vi "Lichen Analysis.vi"(0 "Parameters (Rejilla)":T2(array[cluster])=[{"Name"="Rectangle 1", "Type"=enum."Rotated Rectangle", "Coordinates"=[0, 0, 80, 76, 0], "Colors"=[16711680], "Drawing Mode"=0, "Text"="Your Text", "Results"=[], "Font, Size & Style"={"Desired Font (Application)"=enum."System Font", "[User-specified Font]"={"Font Name"="Tahoma", "Size"=13, "Strikeout?"=FALSE, "Italic?"=FALSE, "Underline?"=FALSE, "Outline?"=FALSE, "Shadow?"=FALSE, "Bold?"=FALSE, "Rotation Angle"=0.0}, "Horizontal Alignment"=0, "Vertical Alignment"=0}, "Image File Path"=path "", "Use Keying Color"=FALSE}, {"Name"="Rectangle 2", "Type"=enum."Rotated Rectangle", "Coordinates"=[81, 0, 161, 76, 0], "Colors"=[16717824], "Drawing Mode"=0, "Text"="Your Text", "Results"=[], "Font, Size & Style"={"Desired Font (Application)"=enum."System Font", "[User-specified Font]"={"Font Name"="Tahoma", "Size"=13, "Strikeout?"=FALSE, "Italic?"=FALSE, "Underline?"=FALSE, "Outline?"=FALSE, "Shadow?"=FALSE, "Bold?"=FALSE, "Rotation Angle"=0.0}, "Horizontal Alignment"=0, "Vertical Alignment"=0}, "Image File Path"=path "", "Use Keying Color"=FALSE}, {"Name"="Rectangle 3", "Type"=enum."Rotated Rectangle", "Coordinates"=[0, 77, 80, 152, 0], "Colors"=[16717824], "Drawing Mode"=0, "Text"="Your Text", "Results"=[], "Font, Size & Style"={"Desired Font (Application)"=enum."System Font", "[User-specified Font]"={"Font Name"="Tahoma", "Size"=13, "Strikeout?"=FALSE, "Italic?"=FALSE, "Underline?"=FALSE, "Outline?"=FALSE, "Shadow?"=FALSE, "Bold?"=FALSE, "Rotation Angle"=0.0}, "Horizontal Alignment"=0, "Vertical Alignment"=0}, "Image File Path"=path "", "Use Keying Color"=FALSE}, {"Name"="Rectangle 4", "Type"=enum."Rotated Rectangle", "Coordinates"=[81, 77, 161, 152, 0], "Colors"=[16717824], "Drawing Mode"=0, "Text"="Your Text", "Results"=[], "Font, Size & Style"={"Desired Font (Application)"=enum."System Font", "[User-specified Font]"={"Font Name"="Tahoma", "Size"=13, "Strikeout?"=FALSE, "Italic?"=FALSE, "Underline?"=FALSE, "Outline?"=FALSE, "Shadow?"=FALSE, "Bold?"=FALSE, "Rotation Angle"=0.0}, "Horizontal Alignment"=0, "Vertical Alignment"=0}, "Image File Path"=path "", "Use Keying Color"=FALSE}, {"Name"="Rectangle 5", "Type"=enum."Rotated Rectangle", "Coordinates"=[0, 153, 80, 228, 0], "Colors"=[16717824], "Drawing Mode"=0, "Text"="Your Text", "Results"=[], "Font, Size & Style"={"Desired Font (Application)"=enum."System Font", "[User-specified Font]"={"Font Name"="Tahoma", "Size"=13, "Strikeout?"=FALSE, "Italic?"=FALSE, "Underline?"=FALSE, "Outline?"=FALSE, "Shadow?"=FALSE, "Bold?"=FALSE, "Rotation Angle"=0.0}, "Horizontal Alignment"=0, "Vertical Alignment"=0}, "Image File Path"=path "", "Use Keying Color"=FALSE}, {"Name"="Rectangle 6", "Type"=enum."Rotated Rectangle", "Coordinates"=[81, 153, 161, 228, 0], "Colors"=[16717824], "Drawing Mode"=0, "Text"="Your Text", "Results"=[], "Font, Size & Style"={"Desired Font (Application)"=enum."System Font", "[User-specified Font]"={"Font Name"="Tahoma", "Size"=13, "Strikeout?"=FALSE, "Italic?"=FALSE, "Underline?"=FALSE, "Outline?"=FALSE, "Shadow?"=FALSE, "Bold?"=FALSE, "Rotation Angle"=0.0}, "Horizontal Alignment"=0, "Vertical Alignment"=0}, "Image File Path"=path "", "Use Keying Color"=FALSE}, {"Name"="Text 1", "Type"=enum."Text", "Coordinates"=[3, 73], "Colors"=[2817810, 16777216], "Drawing Mode"=0, "Text"="Cell 1", "Results"=[], "Font, Size & Style"={"Desired Font (Application)"=enum."System Font", "[User-specified Font]"={"Font Name"="Tahoma", "Size"=13, "Strikeout?"=FALSE, "Italic?"=FALSE, "Underline?"=FALSE, "Outline?"=FALSE, "Shadow?"=FALSE, "Bold?"=FALSE, "Rotation Angle"=0.0}, "Horizontal Alignment"=0, "Vertical Alignment"=0}, "Image File Path"=path "", "Use Keying Color"=FALSE}, {"Name"="Text 2", "Type"=enum."Text", "Coordinates"=[83, 73], "Colors"=[2817810, 16777216], "Drawing Mode"=0, "Text"="Cell 2", "Results"=[], "Font, Size & Style"={"Desired Font (Application)"=enum."System Font", "[User-specified Font]"={"Font Name"="Tahoma", "Size"=13, "Strikeout?"=FALSE, "Italic?"=FALSE, "Underline?"=FALSE, "Outline?"=FALSE, "Shadow?"=FALSE, "Bold?"=FALSE, "Rotation Angle"=0.0}, "Horizontal Alignment"=0, "Vertical Alignment"=0}, "Image File Path"=path "", "Use Keying Color"=FALSE}, {"Name"="Text 3", "Type"=enum."Text", "Coordinates"=[3, 149], "Colors"=[2817810, 16777216], "Drawing Mode"=0, "Text"="Cell 3", "Results"=[], "Font, Size & Style"={"Desired Font (Application)"=enum."System Font", "[User-specified Font]"={"Font Name"="Tahoma", "Size"=13, "Strikeout?"=FALSE, "Italic?"=FALSE, "Underline?"=FALSE, "Outline?"=FALSE, "Shadow?"=FALSE, "Bold?"=FALSE, "Rotation Angle"=0.0}, "Horizontal Alignment"=0, "Vertical Alignment"=0}, "Image File Path"=path "", "Use Keying Color"=FALSE}, {"Name"="Text 4", "Type"=enum."Text", "Coordinates"=[83, 149], "Colors"=[2817810, 16777216], "Drawing Mode"=0, "Text"="Cell 4", "Results"=[], "Font, Size & Style"={"Desired Font (Application)"=enum."System Font", "[User-specified Font]"={"Font Name"="Tahoma", "Size"=13, "Strikeout?"=FALSE, "Italic?"=FALSE, "Underline?"=FALSE, "Outline?"=FALSE, "Shadow?"=FALSE, "Bold?"=FALSE, "Rotation Angle"=0.0}, "Horizontal Alignment"=0, "Vertical Alignment"=0}, "Image File Path"=path "", "Use Keying Color"=FALSE}, {"Name"="Text 5", "Type"=enum."Text", "Coordinates"=[3, 225], "Colors"=[2817810, 16777216], "Drawing Mode"=0, "Text"="Cell 5", "Results"=[], "Font, Size & Style"={"Desired Font (Application)"=enum."System Font", "[User-specified Font]"={"Font Name"="Tahoma", "Size"=13, "Strikeout?"=FALSE, "Italic?"=FALSE, "Underline?"=FALSE, "Outline?"=FALSE, "Shadow?"=FALSE, "Bold?"=FALSE, "Rotation Angle"=0.0}, "Horizontal Alignment"=0, "Vertical Alignment"=0}, "Image File Path"=path "", "Use Keying Color"=FALSE}, {"Name"="Text 6", "Type"=enum."Text", "Coordinates"=[83, 225], "Colors"=[65407, 16777216], "Drawing Mode"=0, "Text"="Cell 6", "Results"=[], "Font, Size & Style"={"Desired Font (Application)"=enum."System Font", "[User-specified Font]"={"Font Name"="Tahoma", "Size"=13, "Strikeout?"=FALSE, "Italic?"=FALSE, "Underline?"=FALSE, "Outline?"=FALSE, "Shadow?"=FALSE, "Bold?"=FALSE, "Rotation Angle"=0.0}, "Horizontal Alignment"=0, "Vertical Alignment"=0}, "Image File Path"=path "", "Use Keying Color"=FALSE}] {"Drawing Mode" items=["Frame", "Fill", "Highlight"]; "Results"."String Format" items=["Decimal", "Hexadecimal", "Octal", "Fractional", "Exponential", "Engineering"]; "Font, Size & Style"."Horizontal Alignment" items=["Left", "Center", "Right"]; "Font, Size & Style"."Vertical Alignment" items=["Bottom", "Top", "Baseline"]}, 1 "ROI Descriptor (Lichen 1 Cell 1)":T1={"Global Rectangle"=[1, 0, 80, 76], "Contours"=[{"ID"=enum."External", "Type"=12, "Coordinates"=[1, 0, 80, 76, 0]}]} {"Contours"."Type" items=["No Selection", "Point", "Line", "Rectangle", "Oval", "Polygon", "Freehand Region", "Annulus", "Unused2", "Unused3", "Broken Line", "Freehand Line", "Rotated Rectangle"]}, 2 "ROI Descriptor (Lichen 1 Cell 2)":T1={"Global Rectangle"=[81, 0, 161, 76], "Contours"=[{"ID"=enum."External", "Type"=12, "Coordinates"=[81, 0, 161, 76, 0]}]} {"Contours"."Type" items=["No Selection", "Point", "Line", "Rectangle", "Oval", "Polygon", "Freehand Region", "Annulus", "Unused2", "Unused3", "Broken Line", "Freehand Line", "Rotated Rectangle"]}, 3 "ROI Descriptor (Lichen 1 Cell 3)":T1={"Global Rectangle"=[0, 77, 80, 152], "Contours"=[{"ID"=enum."External", "Type"=12, "Coordinates"=[0, 77, 80, 152, 0]}]} {"Contours"."Type" items=["No Selection", "Point", "Line", "Rectangle", "Oval", "Polygon", "Freehand Region", "Annulus", "Unused2", "Unused3", "Broken Line", "Freehand Line", "Rotated Rectangle"]}, 4 "ROI Descriptor (Lichen 1 Cell 4)":T1={"Global Rectangle"=[81, 77, 161, 152], "Contours"=[{"ID"=enum."External", "Type"=12, "Coordinates"=[81, 77, 161, 152, 0]}]} {"Contours"."Type" items=["No Selection", "Point", "Line", "Rectangle", "Oval", "Polygon", "Freehand Region", "Annulus", "Unused2", "Unused3", "Broken Line", "Freehand Line", "Rotated Rectangle"]}, 5 "ROI Descriptor (Lichen 1 Cell 5)":T1={"Global Rectangle"=[0, 153, 80, 228], "Contours"=[{"ID"=enum."External", "Type"=12, "Coordinates"=[0, 153, 80, 228, 0]}]} {"Contours"."Type" items=["No Selection", "Point", "Line", "Rectangle", "Oval", "Polygon", "Freehand Region", "Annulus", "Unused2", "Unused3", "Broken Line", "Freehand Line", "Rotated Rectangle"]}, 6 "ROI Descriptor (Lichen 1 Cell 6)":T1={"Global Rectangle"=[81, 153, 161, 228], "Contours"=[{"ID"=enum."External", "Type"=12, "Coordinates"=[81, 153, 161, 228, 0]}]} {"Contours"."Type" items=["No Selection", "Point", "Line", "Rectangle", "Oval", "Polygon", "Freehand Region", "Annulus", "Unused2", "Unused3", "Broken Line", "Freehand Line", "Rotated Rectangle"]}, 7 "error in":errorcluster, 8 "ROI Descriptor (Lichen 2 Cell1)":T1={"Global Rectangle"=[0, 0, 80, 76], "Contours"=[{"ID"=enum."External", "Type"=12, "Coordinates"=[0, 0, 80, 76, 0]}]} {"Contours"."Type" items=["No Selection", "Point", "Line", "Rectangle", "Oval", "Polygon", "Freehand Region", "Annulus", "Unused2", "Unused3", "Broken Line", "Freehand Line", "Rotated Rectangle"]}, 9 "ROI Descriptor (Lichen 2 Cell 2)":T1={"Global Rectangle"=[81, 0, 161, 76], "Contours"=[{"ID"=enum."External", "Type"=12, "Coordinates"=[81, 0, 161, 76, 0]}]} {"Contours"."Type" items=["No Selection", "Point", "Line", "Rectangle", "Oval", "Polygon", "Freehand Region", "Annulus", "Unused2", "Unused3", "Broken Line", "Freehand Line", "Rotated Rectangle"]}, 10 "ROI Descriptor (Lichen 2 Cell 3)":T1={"Global Rectangle"=[0, 77, 80, 152], "Contours"=[{"ID"=enum."External", "Type"=12, "Coordinates"=[0, 77, 80, 152, 0]}]} {"Contours"."Type" items=["No Selection", "Point", "Line", "Rectangle", "Oval", "Polygon", "Freehand Region", "Annulus", "Unused2", "Unused3", "Broken Line", "Freehand Line", "Rotated Rectangle"]}, 11 "ROI Descriptor (Lichen 2 Cell 4)":T1={"Global Rectangle"=[81, 77, 161, 152], "Contours"=[{"ID"=enum."External", "Type"=12, "Coordinates"=[81, 77, 161, 152, 0]}]} {"Contours"."Type" items=["No Selection", "Point", "Line", "Rectangle", "Oval", "Polygon", "Freehand Region", "Annulus", "Unused2", "Unused3", "Broken Line", "Freehand Line", "Rotated Rectangle"]}, 12 "ROI Descriptor (Lichen 2 Cell 5)":T1={"Global Rectangle"=[0, 153, 80, 228], "Contours"=[{"ID"=enum."External", "Type"=12, "Coordinates"=[0, 153, 80, 228, 0]}]} {"Contours"."Type" items=["No Selection", "Point", "Line", "Rectangle", "Oval", "Polygon", "Freehand Region", "Annulus", "Unused2", "Unused3", "Broken Line", "Freehand Line", "Rotated Rectangle"]}, 13 "ROI Descriptor (Lichen 2 Cell 6)":T1={"Global Rectangle"=[81, 153, 161, 228], "Contours"=[{"ID"=enum."External", "Type"=12, "Coordinates"=[81, 153, 161, 228, 0]}]} {"Contours"."Type" items=["No Selection", "Point", "Line", "Rectangle", "Oval", "Polygon", "Freehand Region", "Annulus", "Unused2", "Unused3", "Broken Line", "Freehand Line", "Rotated Rectangle"]}) -> (14 "Histogram (Histogram 2)":u32[][](array[numeric]), 15 "Number of Matches (Lichen 2 Cell 6)":i32, 16 "Number of Matches (Lichen 2 Cell 5)":i32, 17 "Number of Matches (Lichen 2 Cell 4)":i32, 18 "Number of Matches (Lichen 2 Cell 3)":i32, 19 "Number of Matches (Lichen 2 Cell 2)":i32, 20 "Number of Matches (Lichen 1 Cell 1)":i32, 21 "Number of Matches (Lichen 1 Cell 2)":i32, 22 "Number of Matches (Lichen 1 Cell 3)":i32, 23 "Number of Matches (Lichen 1 Cell 4)":i32, 24 "Number of Matches (Lichen 1 Cell 5)":i32, 25 "Number of Matches (Lichen 1 Cell 6)":i32, 26 "Number of Matches (Lichen 2 Cell1)":i32, 27 "error out":errorcluster)   [LabVIEW 2018]
uses:
  <vilib>/vision/NI_Vision_Development_Module.lvlib
panel:
  out "Image Out":T3(plugin-control)
  out "Histogram Graph 2":u32[][](graph)
  out "Histogram Graph":u32[][](graph)
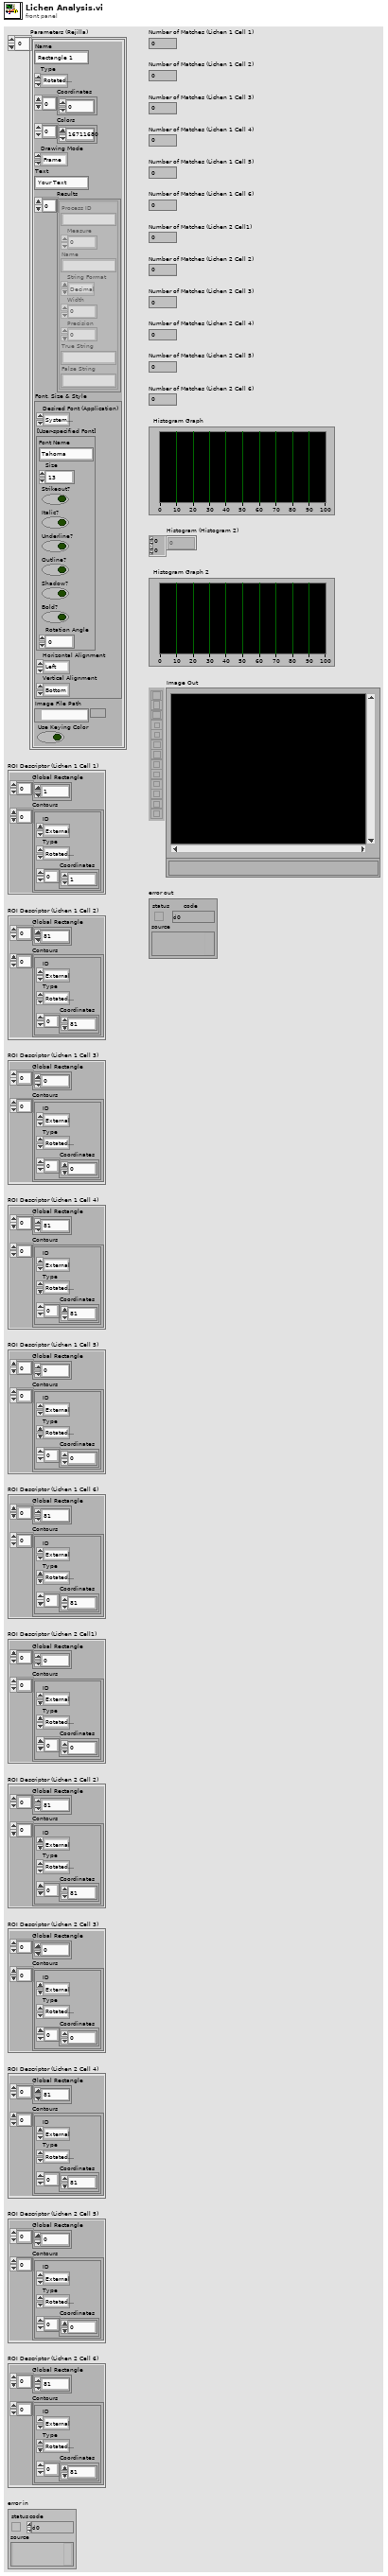
[diagram p1: front panel]
types:
  T1 = cluster{"Global Rectangle":i32[], "Contours":cluster{"ID":enum32{"External", "Internal"}, "Type":u32, "Coordinates":i32[]}[]}
  T2 = cluster{"Name":string, "Type":enum16{"Line", "Broken Line", "Free Hand Line", "Rotated Rectangle", "Oval", "Polygon", "Free Hand", "Bitmap", "Text"}, "Coordinates":i32[], "Colors":u32[], "Drawing Mode":u32, "Text":string, "Results":cluster{"Process ID":string, "Measure":u16, "Name":string, "String Format":u16, "Width":i16, "Precision":i16, "True String":string, "False String":string}[], "Font, Size & Style":cluster{"Desired Font (Application)":enum16{"User-specified Font", "Application Font", "System Font", "Dialog Font"}, "[User-specified Font]":cluster{"Font Name":string, "Size":i16, "Strikeout?":bool, "Italic?":bool, "Underline?":bool, "Outline?":bool, "Shadow?":bool, "Bold?":bool, "Rotation Angle":dbl}, "Horizontal Alignment":i16, "Vertical Alignment":i16}, "Image File Path":path, "Use Keying Color":bool}[]
  T3 = typedef "IMAQ Image.ctl" = refnum<image>
  T4 = typedef "Image Type" = u32
  T5 = cluster{"Position":cluster{"x":sgl, "y":sgl}, "Angle":sgl, "Scale":sgl, "Score":sgl, "Bounding Box":cluster{"x":sgl, "y":sgl}[]}[]
diagram:
  w1 = u32 1 items=["Grayscale", "Binary", "Gradient", "Rainbow", "Temperature", "User Defined", "Binary 16 Bit", "Gradient 16 Bit", "Rainbow 16 Bit", "Temperature 16 Bit", "User Defined 16 Bit"] ("Palette Type")
  w10 = u16 0 items=["RGB", "HSL", "HSV", "HSI"] ("Color Mode")
  w8 = T1 {"Global Rectangle"=[-10, 0, 161, 234], "Contours"=[{"ID"=enum."External", "Type"=3, "Coordinates"=[-10, 0, 161, 234]}]}  # ROI Descriptor
  w18 = u16 1 items=["RGB", "HSL", "HSV", "HSI"] ("Color Mode")
  w27 = 10  # Bit Depth
  w28 = FALSE  # Set Bit Depth
  w37 = u16 0 items=["RGB", "HSL", "HSV", "HSI"] ("Color Mode")
  w35 = T1 {"Global Rectangle"=[0, 0, 161, 228], "Contours"=[{"ID"=enum."External", "Type"=3, "Coordinates"=[0, 0, 161, 228]}]}  # ROI Descriptor
  w54 = u16 0 items=["RGB", "HSL", "HSV", "HSI"] ("Color Mode")
  w63 = "Lichen 2 Cell 6" ("Step Name")
  w68 = T4 4 items=["Grayscale (U8)", "Grayscale (I16)", "Grayscale (SGL)", "Complex (CSG)", "RGB (U32)", "HSL (U32)", "RGB (U64)"] ("Image Type")
  w70 = u32 1 items=["Conservative", "Balance", "Aggressive", "Very Aggressive"] ("Search Strategy")
  w71 = u32 0 items=["Low Sensitivity", "Medium Sensitivity", "High Sensitivity"] ("Color Sensitivity")
  w72 = u32 1 items=["Color and Shape", "Color", "Shape"] ("Match Feature Mode")
  w83 = "Lichen 2 Cell 5" ("Step Name")
  w88 = T4 4 items=["Grayscale (U8)", "Grayscale (I16)", "Grayscale (SGL)", "Complex (CSG)", "RGB (U32)", "HSL (U32)", "RGB (U64)"] ("Image Type")
  w90 = u32 1 items=["Conservative", "Balance", "Aggressive", "Very Aggressive"] ("Search Strategy")
  w91 = u32 0 items=["Low Sensitivity", "Medium Sensitivity", "High Sensitivity"] ("Color Sensitivity")
  w92 = u32 1 items=["Color and Shape", "Color", "Shape"] ("Match Feature Mode")
  w103 = "Lichen 2 Cell 4" ("Step Name")
  w108 = T4 4 items=["Grayscale (U8)", "Grayscale (I16)", "Grayscale (SGL)", "Complex (CSG)", "RGB (U32)", "HSL (U32)", "RGB (U64)"] ("Image Type")
  w110 = u32 0 items=["Conservative", "Balance", "Aggressive", "Very Aggressive"] ("Search Strategy")
  w111 = u32 0 items=["Low Sensitivity", "Medium Sensitivity", "High Sensitivity"] ("Color Sensitivity")
  w112 = u32 1 items=["Color and Shape", "Color", "Shape"] ("Match Feature Mode")
  w123 = "Lichen 2 Cell 3" ("Step Name")
  w128 = T4 4 items=["Grayscale (U8)", "Grayscale (I16)", "Grayscale (SGL)", "Complex (CSG)", "RGB (U32)", "HSL (U32)", "RGB (U64)"] ("Image Type")
  w130 = u32 0 items=["Conservative", "Balance", "Aggressive", "Very Aggressive"] ("Search Strategy")
  w131 = u32 0 items=["Low Sensitivity", "Medium Sensitivity", "High Sensitivity"] ("Color Sensitivity")
  w132 = u32 1 items=["Color and Shape", "Color", "Shape"] ("Match Feature Mode")
  w143 = "Lichen 2 Cell 2" ("Step Name")
  w148 = T4 4 items=["Grayscale (U8)", "Grayscale (I16)", "Grayscale (SGL)", "Complex (CSG)", "RGB (U32)", "HSL (U32)", "RGB (U64)"] ("Image Type")
  w150 = u32 2 items=["Conservative", "Balance", "Aggressive", "Very Aggressive"] ("Search Strategy")
  w151 = u32 0 items=["Low Sensitivity", "Medium Sensitivity", "High Sensitivity"] ("Color Sensitivity")
  w152 = u32 1 items=["Color and Shape", "Color", "Shape"] ("Match Feature Mode")
  w163 = "Lichen 2 Cell1" ("Step Name")
  w168 = T4 4 items=["Grayscale (U8)", "Grayscale (I16)", "Grayscale (SGL)", "Complex (CSG)", "RGB (U32)", "HSL (U32)", "RGB (U64)"] ("Image Type")
  w170 = u32 2 items=["Conservative", "Balance", "Aggressive", "Very Aggressive"] ("Search Strategy")
  w171 = u32 0 items=["Low Sensitivity", "Medium Sensitivity", "High Sensitivity"] ("Color Sensitivity")
  w172 = u32 1 items=["Color and Shape", "Color", "Shape"] ("Match Feature Mode")
  w183 = "Lichen 1 Cell 6" ("Step Name")
  w188 = T4 4 items=["Grayscale (U8)", "Grayscale (I16)", "Grayscale (SGL)", "Complex (CSG)", "RGB (U32)", "HSL (U32)", "RGB (U64)"] ("Image Type")
  w190 = u32 0 items=["Conservative", "Balance", "Aggressive", "Very Aggressive"] ("Search Strategy")
  w191 = u32 0 items=["Low Sensitivity", "Medium Sensitivity", "High Sensitivity"] ("Color Sensitivity")
  w192 = u32 1 items=["Color and Shape", "Color", "Shape"] ("Match Feature Mode")
  w203 = "Lichen 1 Cell 5" ("Step Name")
  w208 = T4 4 items=["Grayscale (U8)", "Grayscale (I16)", "Grayscale (SGL)", "Complex (CSG)", "RGB (U32)", "HSL (U32)", "RGB (U64)"] ("Image Type")
  w210 = u32 0 items=["Conservative", "Balance", "Aggressive", "Very Aggressive"] ("Search Strategy")
  w211 = u32 0 items=["Low Sensitivity", "Medium Sensitivity", "High Sensitivity"] ("Color Sensitivity")
  w212 = u32 1 items=["Color and Shape", "Color", "Shape"] ("Match Feature Mode")
  w223 = "Lichen 1 Cell 4" ("Step Name")
  w228 = T4 4 items=["Grayscale (U8)", "Grayscale (I16)", "Grayscale (SGL)", "Complex (CSG)", "RGB (U32)", "HSL (U32)", "RGB (U64)"] ("Image Type")
  w230 = u32 0 items=["Conservative", "Balance", "Aggressive", "Very Aggressive"] ("Search Strategy")
  w231 = u32 0 items=["Low Sensitivity", "Medium Sensitivity", "High Sensitivity"] ("Color Sensitivity")
  w232 = u32 1 items=["Color and Shape", "Color", "Shape"] ("Match Feature Mode")
  w243 = "Lichen 1 Cell 3" ("Step Name")
  w248 = T4 4 items=["Grayscale (U8)", "Grayscale (I16)", "Grayscale (SGL)", "Complex (CSG)", "RGB (U32)", "HSL (U32)", "RGB (U64)"] ("Image Type")
  w250 = u32 0 items=["Conservative", "Balance", "Aggressive", "Very Aggressive"] ("Search Strategy")
  w251 = u32 0 items=["Low Sensitivity", "Medium Sensitivity", "High Sensitivity"] ("Color Sensitivity")
  w252 = u32 1 items=["Color and Shape", "Color", "Shape"] ("Match Feature Mode")
  w263 = "Lichen 1 Cell 2" ("Step Name")
  w268 = T4 4 items=["Grayscale (U8)", "Grayscale (I16)", "Grayscale (SGL)", "Complex (CSG)", "RGB (U32)", "HSL (U32)", "RGB (U64)"] ("Image Type")
  w270 = u32 0 items=["Conservative", "Balance", "Aggressive", "Very Aggressive"] ("Search Strategy")
  w271 = u32 0 items=["Low Sensitivity", "Medium Sensitivity", "High Sensitivity"] ("Color Sensitivity")
  w272 = u32 1 items=["Color and Shape", "Color", "Shape"] ("Match Feature Mode")
  w283 = "Lichen 1 Cell 1" ("Step Name")
  w288 = T4 4 items=["Grayscale (U8)", "Grayscale (I16)", "Grayscale (SGL)", "Complex (CSG)", "RGB (U32)", "HSL (U32)", "RGB (U64)"] ("Image Type")
  w290 = u32 0 items=["Conservative", "Balance", "Aggressive", "Very Aggressive"] ("Search Strategy")
  w291 = u32 0 items=["Low Sensitivity", "Medium Sensitivity", "High Sensitivity"] ("Color Sensitivity")
  w292 = u32 1 items=["Color and Shape", "Color", "Shape"] ("Match Feature Mode")
  w299 = T4 4 items=["Grayscale (U8)", "Grayscale (I16)", "Grayscale (SGL)", "Complex (CSG)", "RGB (U32)", "HSL (U32)", "RGB (U64)", "Grayscale (U16)"] ("Image Type")
  n1 = Call Chain() -> (call chain=w303:string[])
  n2 = Index Array(array=w303) -> (element=w302:string)  [unwired: 1 in]
  n3 = call "File Dialog"("prompt"="Select an image file...") -> ("selected path"=w300:path)  [unwired: 6 in, 8 out]
  n4 = call "IMAQ Create"("Image Name"=w302, "Image Type"=w299, "error in (no error)"="error in") -> ("New Image"=w306:T3, "error out"=w305:errorcluster)  [unwired: 1 in, 1 out]
  n5 = call "IMAQ ReadFile"("File Path"=w300, "error in (no error)"=w305, "Image"=w306) -> ("error out"=w307:errorcluster, "Image Out"=w298:T3)  [unwired: 2 in, 5 out]
  n6 = call <vilib>:"IVA Overlay - Overlay.vi"("error in (no error)"=w307, "Parameters"="Parameters (Rejilla)", "Image In"=w298) -> ("error out"=w297:errorcluster, "Image Out"=w285:T3)  [unwired: 7 out]
  n7 = while {
    shift-right: [w319] -> w279
    shift-left: _ -> [w318]
    tunnel: [w316] -> w278
    tunnel: w297 -> [w315]
    tunnel: path "C:/Users/anton/Desktop/liquenes/lichen1.png" ("File Path") -> [w311]
    tunnel: w288 -> [w314]
    tunnel: w283 -> [w313]
    shift-right: [w311] -> _
    shift-left: _ -> [w312]
    stop <- FALSE continue-if-true
    n8 = First Call?() -> (First Call?: T/F=w310:bool)
    n9 = Not Equal?(x=w312, y=w311) -> (x != y?=w309:bool)
    n10 = Or(x=w309, y=w310) -> (x .or. y?=w308:bool)
    n11 = case shown="True" w308 {
      tunnel: [w321 w334] -> w319
      tunnel: w318 -> [w321 w326]
      tunnel: [w320 w331] -> w316
      tunnel: w315 -> [w320 w325]
      tunnel: w314 -> [_ w330]
      tunnel: w313 -> [_ w327]
      tunnel: w311 -> [_ w323]
      frame False {
      }
      frame True {
        n12 = Call Chain() -> (call chain=w329:string[])
        n13 = stacked-sequence {
          tunnel: w326 -> [w339]
          tunnel: w325 -> [w338]
          tunnel: [w338] -> w324
          tunnel: [w337] -> _
          frame #0 {
            n14 = call "IMAQ Dispose"("Image"=w339) -> ("error out"=w337:errorcluster)  [unwired: 2 in, 3 out]
          }
        }
        n15 = Index Array(array=w329) -> (element=w328:string)  [unwired: 1 in]
        n16 = Format Into String(format string="CL Template %s %s" ("Image Name"), w328, w327) -> (resulting string=w336:string)  [unwired: 2 in, 1 out]
        n17 = call "IMAQ Create"("Image Name"=w336, "Image Type"=w330, "error in (no error)"=w324) -> ("New Image"=w333:T3, "error out"=w332:errorcluster)  [unwired: 1 in, 1 out]
        n18 = call <vilib>:"IVA Get Alternate Path.vi"("Path In"=w323) -> ("Path Out"=w322:path)  [unwired: 10 out]
        n19 = call "IMAQ Read Image And Vision Info"("File Path"=w322, "error in (no error)"=w332, "Image"=w333) -> ("error out"=w331:errorcluster, "Image Out"=w334:T3)  [unwired: 1 in, 6 out]
      }
    }
  }
  n20 = call <vilib>:"IVA Get Alternate Path.vi"("Path In"=path "C:/Users/anton/Desktop/liquenes/test1.jpg" ("File Path")) -> ("Path Out"=w23:path)  [unwired: 10 out]
  n21 = Unbundle By Name("ROI Descriptor (Lichen 1 Cell 1)") -> ("Global Rectangle"=w280:i32[])
  n22 = call "IMAQ Setup Match Color Pattern"("Match Feature Mode"=w292, "error in (no error)"=w278, "Color Sensitivity"=w291, "Search Strategy"=w290) -> ("Match Color Pattern Setup Data"=w282:string, "error out"=w281:errorcluster)  [unwired: 5 in, 5 out]
  n23 = call "IMAQ Match Color Pattern"("Minimum Match Score"=sgl 700.0, "Number of Matches Requested"=1, "Optional Rectangle"=w280, "error in (no error)"=w281, "Match Color Pattern Setup Data"=w282, "Template Image"=w279, "Image"=w285) -> ("error out"=w286:errorcluster, "Number of Matches"=→"Number of Matches (Lichen 1 Cell 1)":i32, "Matches"=w284:T5)  [unwired: 2 out]
  n24 = call <vilib>:"IVA Store Color Location Results.vi"("error in (no error)"=w286, "Matches"=w284, "Step Name"=w283, "Image in"=w285) -> ("error out"=w277:errorcluster, "Image dup"=w265:T3)  [unwired: 6 out]
  n25 = call <vilib>:"IVA Clear Coordsys Errors.vi"("error in (no error)"=w277) -> ("error out"=w276:errorcluster)  [unwired: 10 in]
  n26 = while {
    shift-right: [w351] -> w259
    shift-left: _ -> [w350]
    tunnel: [w348] -> w258
    tunnel: w276 -> [w347]
    tunnel: path "C:/Users/anton/Desktop/liquenes/lichen1.png" ("File Path") -> [w343]
    tunnel: w268 -> [w346]
    tunnel: w263 -> [w345]
    shift-right: [w343] -> _
    shift-left: _ -> [w344]
    stop <- FALSE continue-if-true
    n27 = First Call?() -> (First Call?: T/F=w342:bool)
    n28 = Not Equal?(x=w344, y=w343) -> (x != y?=w341:bool)
    n29 = Or(x=w341, y=w342) -> (x .or. y?=w340:bool)
    n30 = case shown="True" w340 {
      tunnel: [w353 w366] -> w351
      tunnel: w350 -> [w353 w358]
      tunnel: [w352 w363] -> w348
      tunnel: w347 -> [w352 w357]
      tunnel: w346 -> [_ w362]
      tunnel: w345 -> [_ w359]
      tunnel: w343 -> [_ w355]
      frame False {
      }
      frame True {
        n31 = Call Chain() -> (call chain=w361:string[])
        n32 = stacked-sequence {
          tunnel: w358 -> [w371]
          tunnel: w357 -> [w370]
          tunnel: [w370] -> w356
          tunnel: [w369] -> _
          frame #0 {
            n33 = call "IMAQ Dispose"("Image"=w371) -> ("error out"=w369:errorcluster)  [unwired: 2 in, 3 out]
          }
        }
        n34 = Index Array(array=w361) -> (element=w360:string)  [unwired: 1 in]
        n35 = Format Into String(format string="CL Template %s %s" ("Image Name"), w360, w359) -> (resulting string=w368:string)  [unwired: 2 in, 1 out]
        n36 = call "IMAQ Create"("Image Name"=w368, "Image Type"=w362, "error in (no error)"=w356) -> ("New Image"=w365:T3, "error out"=w364:errorcluster)  [unwired: 1 in, 1 out]
        n37 = call <vilib>:"IVA Get Alternate Path.vi"("Path In"=w355) -> ("Path Out"=w354:path)  [unwired: 10 out]
        n38 = call "IMAQ Read Image And Vision Info"("File Path"=w354, "error in (no error)"=w364, "Image"=w365) -> ("error out"=w363:errorcluster, "Image Out"=w366:T3)  [unwired: 1 in, 6 out]
      }
    }
  }
  n39 = Unbundle By Name("ROI Descriptor (Lichen 1 Cell 2)") -> ("Global Rectangle"=w260:i32[])
  n40 = call "IMAQ Setup Match Color Pattern"("Match Feature Mode"=w272, "error in (no error)"=w258, "Color Sensitivity"=w271, "Search Strategy"=w270) -> ("Match Color Pattern Setup Data"=w262:string, "error out"=w261:errorcluster)  [unwired: 5 in, 5 out]
  n41 = call "IMAQ Match Color Pattern"("Minimum Match Score"=sgl 800.0, "Number of Matches Requested"=1, "Optional Rectangle"=w260, "error in (no error)"=w261, "Match Color Pattern Setup Data"=w262, "Template Image"=w259, "Image"=w265) -> ("error out"=w266:errorcluster, "Number of Matches"=→"Number of Matches (Lichen 1 Cell 2)":i32, "Matches"=w264:T5)  [unwired: 2 out]
  n42 = call <vilib>:"IVA Store Color Location Results.vi"("error in (no error)"=w266, "Matches"=w264, "Step Name"=w263, "Image in"=w265) -> ("error out"=w257:errorcluster, "Image dup"=w245:T3)  [unwired: 6 out]
  n43 = call <vilib>:"IVA Clear Coordsys Errors.vi"("error in (no error)"=w257) -> ("error out"=w256:errorcluster)  [unwired: 10 in]
  n44 = while {
    shift-right: [w383] -> w239
    shift-left: _ -> [w382]
    tunnel: [w380] -> w238
    tunnel: w256 -> [w379]
    tunnel: path "C:/Users/anton/Desktop/liquenes/lichen1.png" ("File Path") -> [w375]
    tunnel: w248 -> [w378]
    tunnel: w243 -> [w377]
    shift-right: [w375] -> _
    shift-left: _ -> [w376]
    stop <- FALSE continue-if-true
    n45 = First Call?() -> (First Call?: T/F=w374:bool)
    n46 = Not Equal?(x=w376, y=w375) -> (x != y?=w373:bool)
    n47 = Or(x=w373, y=w374) -> (x .or. y?=w372:bool)
    n48 = case shown="True" w372 {
      tunnel: [w385 w398] -> w383
      tunnel: w382 -> [w385 w390]
      tunnel: [w384 w395] -> w380
      tunnel: w379 -> [w384 w389]
      tunnel: w378 -> [_ w394]
      tunnel: w377 -> [_ w391]
      tunnel: w375 -> [_ w387]
      frame False {
      }
      frame True {
        n49 = Call Chain() -> (call chain=w393:string[])
        n50 = stacked-sequence {
          tunnel: w390 -> [w403]
          tunnel: w389 -> [w402]
          tunnel: [w402] -> w388
          tunnel: [w401] -> _
          frame #0 {
            n51 = call "IMAQ Dispose"("Image"=w403) -> ("error out"=w401:errorcluster)  [unwired: 2 in, 3 out]
          }
        }
        n52 = Index Array(array=w393) -> (element=w392:string)  [unwired: 1 in]
        n53 = Format Into String(format string="CL Template %s %s" ("Image Name"), w392, w391) -> (resulting string=w400:string)  [unwired: 2 in, 1 out]
        n54 = call "IMAQ Create"("Image Name"=w400, "Image Type"=w394, "error in (no error)"=w388) -> ("New Image"=w397:T3, "error out"=w396:errorcluster)  [unwired: 1 in, 1 out]
        n55 = call <vilib>:"IVA Get Alternate Path.vi"("Path In"=w387) -> ("Path Out"=w386:path)  [unwired: 10 out]
        n56 = call "IMAQ Read Image And Vision Info"("File Path"=w386, "error in (no error)"=w396, "Image"=w397) -> ("error out"=w395:errorcluster, "Image Out"=w398:T3)  [unwired: 1 in, 6 out]
      }
    }
  }
  n57 = Unbundle By Name("ROI Descriptor (Lichen 1 Cell 3)") -> ("Global Rectangle"=w240:i32[])
  n58 = call "IMAQ Setup Match Color Pattern"("Match Feature Mode"=w252, "error in (no error)"=w238, "Color Sensitivity"=w251, "Search Strategy"=w250) -> ("Match Color Pattern Setup Data"=w242:string, "error out"=w241:errorcluster)  [unwired: 5 in, 5 out]
  n59 = call "IMAQ Match Color Pattern"("Minimum Match Score"=sgl 800.0, "Number of Matches Requested"=1, "Optional Rectangle"=w240, "error in (no error)"=w241, "Match Color Pattern Setup Data"=w242, "Template Image"=w239, "Image"=w245) -> ("error out"=w246:errorcluster, "Number of Matches"=→"Number of Matches (Lichen 1 Cell 3)":i32, "Matches"=w244:T5)  [unwired: 2 out]
  n60 = call <vilib>:"IVA Store Color Location Results.vi"("error in (no error)"=w246, "Matches"=w244, "Step Name"=w243, "Image in"=w245) -> ("error out"=w237:errorcluster, "Image dup"=w225:T3)  [unwired: 6 out]
  n61 = call <vilib>:"IVA Clear Coordsys Errors.vi"("error in (no error)"=w237) -> ("error out"=w236:errorcluster)  [unwired: 10 in]
  n62 = while {
    shift-right: [w415] -> w219
    shift-left: _ -> [w414]
    tunnel: [w412] -> w218
    tunnel: w236 -> [w411]
    tunnel: path "C:/Users/anton/Desktop/liquenes/lichen1.png" ("File Path") -> [w407]
    tunnel: w228 -> [w410]
    tunnel: w223 -> [w409]
    shift-right: [w407] -> _
    shift-left: _ -> [w408]
    stop <- FALSE continue-if-true
    n63 = First Call?() -> (First Call?: T/F=w406:bool)
    n64 = Not Equal?(x=w408, y=w407) -> (x != y?=w405:bool)
    n65 = Or(x=w405, y=w406) -> (x .or. y?=w404:bool)
    n66 = case shown="True" w404 {
      tunnel: [w417 w430] -> w415
      tunnel: w414 -> [w417 w422]
      tunnel: [w416 w427] -> w412
      tunnel: w411 -> [w416 w421]
      tunnel: w410 -> [_ w426]
      tunnel: w409 -> [_ w423]
      tunnel: w407 -> [_ w419]
      frame False {
      }
      frame True {
        n67 = Call Chain() -> (call chain=w425:string[])
        n68 = stacked-sequence {
          tunnel: w422 -> [w435]
          tunnel: w421 -> [w434]
          tunnel: [w434] -> w420
          tunnel: [w433] -> _
          frame #0 {
            n69 = call "IMAQ Dispose"("Image"=w435) -> ("error out"=w433:errorcluster)  [unwired: 2 in, 3 out]
          }
        }
        n70 = Index Array(array=w425) -> (element=w424:string)  [unwired: 1 in]
        n71 = Format Into String(format string="CL Template %s %s" ("Image Name"), w424, w423) -> (resulting string=w432:string)  [unwired: 2 in, 1 out]
        n72 = call "IMAQ Create"("Image Name"=w432, "Image Type"=w426, "error in (no error)"=w420) -> ("New Image"=w429:T3, "error out"=w428:errorcluster)  [unwired: 1 in, 1 out]
        n73 = call <vilib>:"IVA Get Alternate Path.vi"("Path In"=w419) -> ("Path Out"=w418:path)  [unwired: 10 out]
        n74 = call "IMAQ Read Image And Vision Info"("File Path"=w418, "error in (no error)"=w428, "Image"=w429) -> ("error out"=w427:errorcluster, "Image Out"=w430:T3)  [unwired: 1 in, 6 out]
      }
    }
  }
  n75 = Unbundle By Name("ROI Descriptor (Lichen 1 Cell 4)") -> ("Global Rectangle"=w220:i32[])
  n76 = call "IMAQ Setup Match Color Pattern"("Match Feature Mode"=w232, "error in (no error)"=w218, "Color Sensitivity"=w231, "Search Strategy"=w230) -> ("Match Color Pattern Setup Data"=w222:string, "error out"=w221:errorcluster)  [unwired: 5 in, 5 out]
  n77 = call "IMAQ Match Color Pattern"("Minimum Match Score"=sgl 800.0, "Number of Matches Requested"=1, "Optional Rectangle"=w220, "error in (no error)"=w221, "Match Color Pattern Setup Data"=w222, "Template Image"=w219, "Image"=w225) -> ("error out"=w226:errorcluster, "Number of Matches"=→"Number of Matches (Lichen 1 Cell 4)":i32, "Matches"=w224:T5)  [unwired: 2 out]
  n78 = call <vilib>:"IVA Store Color Location Results.vi"("error in (no error)"=w226, "Matches"=w224, "Step Name"=w223, "Image in"=w225) -> ("error out"=w217:errorcluster, "Image dup"=w205:T3)  [unwired: 6 out]
  n79 = call <vilib>:"IVA Clear Coordsys Errors.vi"("error in (no error)"=w217) -> ("error out"=w216:errorcluster)  [unwired: 10 in]
  n80 = while {
    shift-right: [w447] -> w199
    shift-left: _ -> [w446]
    tunnel: [w444] -> w198
    tunnel: w216 -> [w443]
    tunnel: path "C:/Users/anton/Desktop/liquenes/lichen1.png" ("File Path") -> [w439]
    tunnel: w208 -> [w442]
    tunnel: w203 -> [w441]
    shift-right: [w439] -> _
    shift-left: _ -> [w440]
    stop <- FALSE continue-if-true
    n81 = First Call?() -> (First Call?: T/F=w438:bool)
    n82 = Not Equal?(x=w440, y=w439) -> (x != y?=w437:bool)
    n83 = Or(x=w437, y=w438) -> (x .or. y?=w436:bool)
    n84 = case shown="True" w436 {
      tunnel: [w449 w462] -> w447
      tunnel: w446 -> [w449 w454]
      tunnel: [w448 w459] -> w444
      tunnel: w443 -> [w448 w453]
      tunnel: w442 -> [_ w458]
      tunnel: w441 -> [_ w455]
      tunnel: w439 -> [_ w451]
      frame False {
      }
      frame True {
        n85 = Call Chain() -> (call chain=w457:string[])
        n86 = stacked-sequence {
          tunnel: w454 -> [w467]
          tunnel: w453 -> [w466]
          tunnel: [w466] -> w452
          tunnel: [w465] -> _
          frame #0 {
            n87 = call "IMAQ Dispose"("Image"=w467) -> ("error out"=w465:errorcluster)  [unwired: 2 in, 3 out]
          }
        }
        n88 = Index Array(array=w457) -> (element=w456:string)  [unwired: 1 in]
        n89 = Format Into String(format string="CL Template %s %s" ("Image Name"), w456, w455) -> (resulting string=w464:string)  [unwired: 2 in, 1 out]
        n90 = call "IMAQ Create"("Image Name"=w464, "Image Type"=w458, "error in (no error)"=w452) -> ("New Image"=w461:T3, "error out"=w460:errorcluster)  [unwired: 1 in, 1 out]
        n91 = call <vilib>:"IVA Get Alternate Path.vi"("Path In"=w451) -> ("Path Out"=w450:path)  [unwired: 10 out]
        n92 = call "IMAQ Read Image And Vision Info"("File Path"=w450, "error in (no error)"=w460, "Image"=w461) -> ("error out"=w459:errorcluster, "Image Out"=w462:T3)  [unwired: 1 in, 6 out]
      }
    }
  }
  n93 = Unbundle By Name("ROI Descriptor (Lichen 1 Cell 5)") -> ("Global Rectangle"=w200:i32[])
  n94 = call "IMAQ Setup Match Color Pattern"("Match Feature Mode"=w212, "error in (no error)"=w198, "Color Sensitivity"=w211, "Search Strategy"=w210) -> ("Match Color Pattern Setup Data"=w202:string, "error out"=w201:errorcluster)  [unwired: 5 in, 5 out]
  n95 = call "IMAQ Match Color Pattern"("Minimum Match Score"=sgl 800.0, "Number of Matches Requested"=1, "Optional Rectangle"=w200, "error in (no error)"=w201, "Match Color Pattern Setup Data"=w202, "Template Image"=w199, "Image"=w205) -> ("error out"=w206:errorcluster, "Number of Matches"=→"Number of Matches (Lichen 1 Cell 5)":i32, "Matches"=w204:T5)  [unwired: 2 out]
  n96 = call <vilib>:"IVA Store Color Location Results.vi"("error in (no error)"=w206, "Matches"=w204, "Step Name"=w203, "Image in"=w205) -> ("error out"=w197:errorcluster, "Image dup"=w185:T3)  [unwired: 6 out]
  n97 = call <vilib>:"IVA Clear Coordsys Errors.vi"("error in (no error)"=w197) -> ("error out"=w196:errorcluster)  [unwired: 10 in]
  n98 = while {
    shift-right: [w479] -> w179
    shift-left: _ -> [w478]
    tunnel: [w476] -> w178
    tunnel: w196 -> [w475]
    tunnel: path "C:/Users/anton/Desktop/liquenes/lichen1.png" ("File Path") -> [w471]
    tunnel: w188 -> [w474]
    tunnel: w183 -> [w473]
    shift-right: [w471] -> _
    shift-left: _ -> [w472]
    stop <- FALSE continue-if-true
    n99 = First Call?() -> (First Call?: T/F=w470:bool)
    n100 = Not Equal?(x=w472, y=w471) -> (x != y?=w469:bool)
    n101 = Or(x=w469, y=w470) -> (x .or. y?=w468:bool)
    n102 = case shown="True" w468 {
      tunnel: [w481 w494] -> w479
      tunnel: w478 -> [w481 w486]
      tunnel: [w480 w491] -> w476
      tunnel: w475 -> [w480 w485]
      tunnel: w474 -> [_ w490]
      tunnel: w473 -> [_ w487]
      tunnel: w471 -> [_ w483]
      frame False {
      }
      frame True {
        n103 = Call Chain() -> (call chain=w489:string[])
        n104 = stacked-sequence {
          tunnel: w486 -> [w499]
          tunnel: w485 -> [w498]
          tunnel: [w498] -> w484
          tunnel: [w497] -> _
          frame #0 {
            n105 = call "IMAQ Dispose"("Image"=w499) -> ("error out"=w497:errorcluster)  [unwired: 2 in, 3 out]
          }
        }
        n106 = Index Array(array=w489) -> (element=w488:string)  [unwired: 1 in]
        n107 = Format Into String(format string="CL Template %s %s" ("Image Name"), w488, w487) -> (resulting string=w496:string)  [unwired: 2 in, 1 out]
        n108 = call "IMAQ Create"("Image Name"=w496, "Image Type"=w490, "error in (no error)"=w484) -> ("New Image"=w493:T3, "error out"=w492:errorcluster)  [unwired: 1 in, 1 out]
        n109 = call <vilib>:"IVA Get Alternate Path.vi"("Path In"=w483) -> ("Path Out"=w482:path)  [unwired: 10 out]
        n110 = call "IMAQ Read Image And Vision Info"("File Path"=w482, "error in (no error)"=w492, "Image"=w493) -> ("error out"=w491:errorcluster, "Image Out"=w494:T3)  [unwired: 1 in, 6 out]
      }
    }
  }
  n111 = Unbundle By Name("ROI Descriptor (Lichen 1 Cell 6)") -> ("Global Rectangle"=w180:i32[])
  n112 = call "IMAQ Setup Match Color Pattern"("Match Feature Mode"=w192, "error in (no error)"=w178, "Color Sensitivity"=w191, "Search Strategy"=w190) -> ("Match Color Pattern Setup Data"=w182:string, "error out"=w181:errorcluster)  [unwired: 5 in, 5 out]
  n113 = call "IMAQ Match Color Pattern"("Minimum Match Score"=sgl 800.0, "Number of Matches Requested"=1, "Optional Rectangle"=w180, "error in (no error)"=w181, "Match Color Pattern Setup Data"=w182, "Template Image"=w179, "Image"=w185) -> ("error out"=w186:errorcluster, "Number of Matches"=→"Number of Matches (Lichen 1 Cell 6)":i32, "Matches"=w184:T5)  [unwired: 2 out]
  n114 = call <vilib>:"IVA Store Color Location Results.vi"("error in (no error)"=w186, "Matches"=w184, "Step Name"=w183, "Image in"=w185) -> ("error out"=w177:errorcluster, "Image dup"=w165:T3)  [unwired: 6 out]
  n115 = call <vilib>:"IVA Clear Coordsys Errors.vi"("error in (no error)"=w177) -> ("error out"=w176:errorcluster)  [unwired: 10 in]
  n116 = while {
    shift-right: [w511] -> w159
    shift-left: _ -> [w510]
    tunnel: [w508] -> w158
    tunnel: w176 -> [w507]
    tunnel: path "C:/Users/anton/Desktop/liquenes/colorlichen2.png" ("File Path") -> [w503]
    tunnel: w168 -> [w506]
    tunnel: w163 -> [w505]
    shift-right: [w503] -> _
    shift-left: _ -> [w504]
    stop <- FALSE continue-if-true
    n117 = First Call?() -> (First Call?: T/F=w502:bool)
    n118 = Not Equal?(x=w504, y=w503) -> (x != y?=w501:bool)
    n119 = Or(x=w501, y=w502) -> (x .or. y?=w500:bool)
    n120 = case shown="True" w500 {
      tunnel: [w513 w526] -> w511
      tunnel: w510 -> [w513 w518]
      tunnel: [w512 w523] -> w508
      tunnel: w507 -> [w512 w517]
      tunnel: w506 -> [_ w522]
      tunnel: w505 -> [_ w519]
      tunnel: w503 -> [_ w515]
      frame False {
      }
      frame True {
        n121 = Call Chain() -> (call chain=w521:string[])
        n122 = stacked-sequence {
          tunnel: w518 -> [w531]
          tunnel: w517 -> [w530]
          tunnel: [w530] -> w516
          tunnel: [w529] -> _
          frame #0 {
            n123 = call "IMAQ Dispose"("Image"=w531) -> ("error out"=w529:errorcluster)  [unwired: 2 in, 3 out]
          }
        }
        n124 = Index Array(array=w521) -> (element=w520:string)  [unwired: 1 in]
        n125 = Format Into String(format string="CL Template %s %s" ("Image Name"), w520, w519) -> (resulting string=w528:string)  [unwired: 2 in, 1 out]
        n126 = call "IMAQ Create"("Image Name"=w528, "Image Type"=w522, "error in (no error)"=w516) -> ("New Image"=w525:T3, "error out"=w524:errorcluster)  [unwired: 1 in, 1 out]
        n127 = call <vilib>:"IVA Get Alternate Path.vi"("Path In"=w515) -> ("Path Out"=w514:path)  [unwired: 10 out]
        n128 = call "IMAQ Read Image And Vision Info"("File Path"=w514, "error in (no error)"=w524, "Image"=w525) -> ("error out"=w523:errorcluster, "Image Out"=w526:T3)  [unwired: 1 in, 6 out]
      }
    }
  }
  n129 = Unbundle By Name("ROI Descriptor (Lichen 2 Cell1)") -> ("Global Rectangle"=w160:i32[])
  n130 = call "IMAQ Setup Match Color Pattern"("Match Feature Mode"=w172, "error in (no error)"=w158, "Color Sensitivity"=w171, "Search Strategy"=w170) -> ("Match Color Pattern Setup Data"=w162:string, "error out"=w161:errorcluster)  [unwired: 5 in, 5 out]
  n131 = call "IMAQ Match Color Pattern"("Minimum Match Score"=sgl 600.0, "Number of Matches Requested"=1, "Optional Rectangle"=w160, "error in (no error)"=w161, "Match Color Pattern Setup Data"=w162, "Template Image"=w159, "Image"=w165) -> ("error out"=w166:errorcluster, "Number of Matches"=→"Number of Matches (Lichen 2 Cell1)":i32, "Matches"=w164:T5)  [unwired: 2 out]
  n132 = call <vilib>:"IVA Store Color Location Results.vi"("error in (no error)"=w166, "Matches"=w164, "Step Name"=w163, "Image in"=w165) -> ("error out"=w157:errorcluster, "Image dup"=w145:T3)  [unwired: 6 out]
  n133 = call <vilib>:"IVA Clear Coordsys Errors.vi"("error in (no error)"=w157) -> ("error out"=w156:errorcluster)  [unwired: 10 in]
  n134 = while {
    shift-right: [w543] -> w139
    shift-left: _ -> [w542]
    tunnel: [w540] -> w138
    tunnel: w156 -> [w539]
    tunnel: path "C:/Users/anton/Desktop/liquenes/colorlichen2.png" ("File Path") -> [w535]
    tunnel: w148 -> [w538]
    tunnel: w143 -> [w537]
    shift-right: [w535] -> _
    shift-left: _ -> [w536]
    stop <- FALSE continue-if-true
    n135 = First Call?() -> (First Call?: T/F=w534:bool)
    n136 = Not Equal?(x=w536, y=w535) -> (x != y?=w533:bool)
    n137 = Or(x=w533, y=w534) -> (x .or. y?=w532:bool)
    n138 = case shown="True" w532 {
      tunnel: [w545 w558] -> w543
      tunnel: w542 -> [w545 w550]
      tunnel: [w544 w555] -> w540
      tunnel: w539 -> [w544 w549]
      tunnel: w538 -> [_ w554]
      tunnel: w537 -> [_ w551]
      tunnel: w535 -> [_ w547]
      frame False {
      }
      frame True {
        n139 = Call Chain() -> (call chain=w553:string[])
        n140 = stacked-sequence {
          tunnel: w550 -> [w563]
          tunnel: w549 -> [w562]
          tunnel: [w562] -> w548
          tunnel: [w561] -> _
          frame #0 {
            n141 = call "IMAQ Dispose"("Image"=w563) -> ("error out"=w561:errorcluster)  [unwired: 2 in, 3 out]
          }
        }
        n142 = Index Array(array=w553) -> (element=w552:string)  [unwired: 1 in]
        n143 = Format Into String(format string="CL Template %s %s" ("Image Name"), w552, w551) -> (resulting string=w560:string)  [unwired: 2 in, 1 out]
        n144 = call "IMAQ Create"("Image Name"=w560, "Image Type"=w554, "error in (no error)"=w548) -> ("New Image"=w557:T3, "error out"=w556:errorcluster)  [unwired: 1 in, 1 out]
        n145 = call <vilib>:"IVA Get Alternate Path.vi"("Path In"=w547) -> ("Path Out"=w546:path)  [unwired: 10 out]
        n146 = call "IMAQ Read Image And Vision Info"("File Path"=w546, "error in (no error)"=w556, "Image"=w557) -> ("error out"=w555:errorcluster, "Image Out"=w558:T3)  [unwired: 1 in, 6 out]
      }
    }
  }
  n147 = Unbundle By Name("ROI Descriptor (Lichen 2 Cell 2)") -> ("Global Rectangle"=w140:i32[])
  n148 = call "IMAQ Setup Match Color Pattern"("Match Feature Mode"=w152, "error in (no error)"=w138, "Color Sensitivity"=w151, "Search Strategy"=w150) -> ("Match Color Pattern Setup Data"=w142:string, "error out"=w141:errorcluster)  [unwired: 5 in, 5 out]
  n149 = call "IMAQ Match Color Pattern"("Minimum Match Score"=sgl 600.0, "Number of Matches Requested"=1, "Optional Rectangle"=w140, "error in (no error)"=w141, "Match Color Pattern Setup Data"=w142, "Template Image"=w139, "Image"=w145) -> ("error out"=w146:errorcluster, "Number of Matches"=→"Number of Matches (Lichen 2 Cell 2)":i32, "Matches"=w144:T5)  [unwired: 2 out]
  n150 = call <vilib>:"IVA Store Color Location Results.vi"("error in (no error)"=w146, "Matches"=w144, "Step Name"=w143, "Image in"=w145) -> ("error out"=w137:errorcluster, "Image dup"=w125:T3)  [unwired: 6 out]
  n151 = call <vilib>:"IVA Clear Coordsys Errors.vi"("error in (no error)"=w137) -> ("error out"=w136:errorcluster)  [unwired: 10 in]
  n152 = while {
    shift-right: [w575] -> w119
    shift-left: _ -> [w574]
    tunnel: [w572] -> w118
    tunnel: w136 -> [w571]
    tunnel: path "C:/Users/anton/Desktop/liquenes/colorlichen2.png" ("File Path") -> [w567]
    tunnel: w128 -> [w570]
    tunnel: w123 -> [w569]
    shift-right: [w567] -> _
    shift-left: _ -> [w568]
    stop <- FALSE continue-if-true
    n153 = First Call?() -> (First Call?: T/F=w566:bool)
    n154 = Not Equal?(x=w568, y=w567) -> (x != y?=w565:bool)
    n155 = Or(x=w565, y=w566) -> (x .or. y?=w564:bool)
    n156 = case shown="True" w564 {
      tunnel: [w577 w590] -> w575
      tunnel: w574 -> [w577 w582]
      tunnel: [w576 w587] -> w572
      tunnel: w571 -> [w576 w581]
      tunnel: w570 -> [_ w586]
      tunnel: w569 -> [_ w583]
      tunnel: w567 -> [_ w579]
      frame False {
      }
      frame True {
        n157 = Call Chain() -> (call chain=w585:string[])
        n158 = stacked-sequence {
          tunnel: w582 -> [w595]
          tunnel: w581 -> [w594]
          tunnel: [w594] -> w580
          tunnel: [w593] -> _
          frame #0 {
            n159 = call "IMAQ Dispose"("Image"=w595) -> ("error out"=w593:errorcluster)  [unwired: 2 in, 3 out]
          }
        }
        n160 = Index Array(array=w585) -> (element=w584:string)  [unwired: 1 in]
        n161 = Format Into String(format string="CL Template %s %s" ("Image Name"), w584, w583) -> (resulting string=w592:string)  [unwired: 2 in, 1 out]
        n162 = call "IMAQ Create"("Image Name"=w592, "Image Type"=w586, "error in (no error)"=w580) -> ("New Image"=w589:T3, "error out"=w588:errorcluster)  [unwired: 1 in, 1 out]
        n163 = call <vilib>:"IVA Get Alternate Path.vi"("Path In"=w579) -> ("Path Out"=w578:path)  [unwired: 10 out]
        n164 = call "IMAQ Read Image And Vision Info"("File Path"=w578, "error in (no error)"=w588, "Image"=w589) -> ("error out"=w587:errorcluster, "Image Out"=w590:T3)  [unwired: 1 in, 6 out]
      }
    }
  }
  n165 = Unbundle By Name("ROI Descriptor (Lichen 2 Cell 3)") -> ("Global Rectangle"=w120:i32[])
  n166 = call "IMAQ Setup Match Color Pattern"("Match Feature Mode"=w132, "error in (no error)"=w118, "Color Sensitivity"=w131, "Search Strategy"=w130) -> ("Match Color Pattern Setup Data"=w122:string, "error out"=w121:errorcluster)  [unwired: 5 in, 5 out]
  n167 = call "IMAQ Match Color Pattern"("Minimum Match Score"=sgl 600.0, "Number of Matches Requested"=2, "Optional Rectangle"=w120, "error in (no error)"=w121, "Match Color Pattern Setup Data"=w122, "Template Image"=w119, "Image"=w125) -> ("error out"=w126:errorcluster, "Number of Matches"=→"Number of Matches (Lichen 2 Cell 3)":i32, "Matches"=w124:T5)  [unwired: 2 out]
  n168 = call <vilib>:"IVA Store Color Location Results.vi"("error in (no error)"=w126, "Matches"=w124, "Step Name"=w123, "Image in"=w125) -> ("error out"=w117:errorcluster, "Image dup"=w105:T3)  [unwired: 6 out]
  n169 = call <vilib>:"IVA Clear Coordsys Errors.vi"("error in (no error)"=w117) -> ("error out"=w116:errorcluster)  [unwired: 10 in]
  n170 = while {
    shift-right: [w607] -> w99
    shift-left: _ -> [w606]
    tunnel: [w604] -> w98
    tunnel: w116 -> [w603]
    tunnel: path "C:/Users/anton/Desktop/liquenes/colorlichen2.png" ("File Path") -> [w599]
    tunnel: w108 -> [w602]
    tunnel: w103 -> [w601]
    shift-right: [w599] -> _
    shift-left: _ -> [w600]
    stop <- FALSE continue-if-true
    n171 = First Call?() -> (First Call?: T/F=w598:bool)
    n172 = Not Equal?(x=w600, y=w599) -> (x != y?=w597:bool)
    n173 = Or(x=w597, y=w598) -> (x .or. y?=w596:bool)
    n174 = case shown="True" w596 {
      tunnel: [w609 w622] -> w607
      tunnel: w606 -> [w609 w614]
      tunnel: [w608 w619] -> w604
      tunnel: w603 -> [w608 w613]
      tunnel: w602 -> [_ w618]
      tunnel: w601 -> [_ w615]
      tunnel: w599 -> [_ w611]
      frame False {
      }
      frame True {
        n175 = Call Chain() -> (call chain=w617:string[])
        n176 = stacked-sequence {
          tunnel: w614 -> [w627]
          tunnel: w613 -> [w626]
          tunnel: [w626] -> w612
          tunnel: [w625] -> _
          frame #0 {
            n177 = call "IMAQ Dispose"("Image"=w627) -> ("error out"=w625:errorcluster)  [unwired: 2 in, 3 out]
          }
        }
        n178 = Index Array(array=w617) -> (element=w616:string)  [unwired: 1 in]
        n179 = Format Into String(format string="CL Template %s %s" ("Image Name"), w616, w615) -> (resulting string=w624:string)  [unwired: 2 in, 1 out]
        n180 = call "IMAQ Create"("Image Name"=w624, "Image Type"=w618, "error in (no error)"=w612) -> ("New Image"=w621:T3, "error out"=w620:errorcluster)  [unwired: 1 in, 1 out]
        n181 = call <vilib>:"IVA Get Alternate Path.vi"("Path In"=w611) -> ("Path Out"=w610:path)  [unwired: 10 out]
        n182 = call "IMAQ Read Image And Vision Info"("File Path"=w610, "error in (no error)"=w620, "Image"=w621) -> ("error out"=w619:errorcluster, "Image Out"=w622:T3)  [unwired: 1 in, 6 out]
      }
    }
  }
  n183 = Unbundle By Name("ROI Descriptor (Lichen 2 Cell 4)") -> ("Global Rectangle"=w100:i32[])
  n184 = call "IMAQ Setup Match Color Pattern"("Match Feature Mode"=w112, "error in (no error)"=w98, "Color Sensitivity"=w111, "Search Strategy"=w110) -> ("Match Color Pattern Setup Data"=w102:string, "error out"=w101:errorcluster)  [unwired: 5 in, 5 out]
  n185 = call "IMAQ Match Color Pattern"("Minimum Match Score"=sgl 600.0, "Number of Matches Requested"=1, "Optional Rectangle"=w100, "error in (no error)"=w101, "Match Color Pattern Setup Data"=w102, "Template Image"=w99, "Image"=w105) -> ("error out"=w106:errorcluster, "Number of Matches"=→"Number of Matches (Lichen 2 Cell 4)":i32, "Matches"=w104:T5)  [unwired: 2 out]
  n186 = call <vilib>:"IVA Store Color Location Results.vi"("error in (no error)"=w106, "Matches"=w104, "Step Name"=w103, "Image in"=w105) -> ("error out"=w97:errorcluster, "Image dup"=w85:T3)  [unwired: 6 out]
  n187 = call <vilib>:"IVA Clear Coordsys Errors.vi"("error in (no error)"=w97) -> ("error out"=w96:errorcluster)  [unwired: 10 in]
  n188 = while {
    shift-right: [w639] -> w79
    shift-left: _ -> [w638]
    tunnel: [w636] -> w78
    tunnel: w96 -> [w635]
    tunnel: path "C:/Users/anton/Desktop/liquenes/colorlichen2.png" ("File Path") -> [w631]
    tunnel: w88 -> [w634]
    tunnel: w83 -> [w633]
    shift-right: [w631] -> _
    shift-left: _ -> [w632]
    stop <- FALSE continue-if-true
    n189 = First Call?() -> (First Call?: T/F=w630:bool)
    n190 = Not Equal?(x=w632, y=w631) -> (x != y?=w629:bool)
    n191 = Or(x=w629, y=w630) -> (x .or. y?=w628:bool)
    n192 = case shown="True" w628 {
      tunnel: [w641 w654] -> w639
      tunnel: w638 -> [w641 w646]
      tunnel: [w640 w651] -> w636
      tunnel: w635 -> [w640 w645]
      tunnel: w634 -> [_ w650]
      tunnel: w633 -> [_ w647]
      tunnel: w631 -> [_ w643]
      frame False {
      }
      frame True {
        n193 = Call Chain() -> (call chain=w649:string[])
        n194 = stacked-sequence {
          tunnel: w646 -> [w659]
          tunnel: w645 -> [w658]
          tunnel: [w658] -> w644
          tunnel: [w657] -> _
          frame #0 {
            n195 = call "IMAQ Dispose"("Image"=w659) -> ("error out"=w657:errorcluster)  [unwired: 2 in, 3 out]
          }
        }
        n196 = Index Array(array=w649) -> (element=w648:string)  [unwired: 1 in]
        n197 = Format Into String(format string="CL Template %s %s" ("Image Name"), w648, w647) -> (resulting string=w656:string)  [unwired: 2 in, 1 out]
        n198 = call "IMAQ Create"("Image Name"=w656, "Image Type"=w650, "error in (no error)"=w644) -> ("New Image"=w653:T3, "error out"=w652:errorcluster)  [unwired: 1 in, 1 out]
        n199 = call <vilib>:"IVA Get Alternate Path.vi"("Path In"=w643) -> ("Path Out"=w642:path)  [unwired: 10 out]
        n200 = call "IMAQ Read Image And Vision Info"("File Path"=w642, "error in (no error)"=w652, "Image"=w653) -> ("error out"=w651:errorcluster, "Image Out"=w654:T3)  [unwired: 1 in, 6 out]
      }
    }
  }
  n201 = Unbundle By Name("ROI Descriptor (Lichen 2 Cell 5)") -> ("Global Rectangle"=w80:i32[])
  n202 = call "IMAQ Setup Match Color Pattern"("Match Feature Mode"=w92, "error in (no error)"=w78, "Color Sensitivity"=w91, "Search Strategy"=w90) -> ("Match Color Pattern Setup Data"=w82:string, "error out"=w81:errorcluster)  [unwired: 5 in, 5 out]
  n203 = call "IMAQ Match Color Pattern"("Minimum Match Score"=sgl 600.0, "Number of Matches Requested"=1, "Optional Rectangle"=w80, "error in (no error)"=w81, "Match Color Pattern Setup Data"=w82, "Template Image"=w79, "Image"=w85) -> ("error out"=w86:errorcluster, "Number of Matches"=→"Number of Matches (Lichen 2 Cell 5)":i32, "Matches"=w84:T5)  [unwired: 2 out]
  n204 = call <vilib>:"IVA Store Color Location Results.vi"("error in (no error)"=w86, "Matches"=w84, "Step Name"=w83, "Image in"=w85) -> ("error out"=w77:errorcluster, "Image dup"=w65:T3)  [unwired: 6 out]
  n205 = call <vilib>:"IVA Clear Coordsys Errors.vi"("error in (no error)"=w77) -> ("error out"=w76:errorcluster)  [unwired: 10 in]
  n206 = while {
    shift-right: [w671] -> w59
    shift-left: _ -> [w670]
    tunnel: [w668] -> w58
    tunnel: w76 -> [w667]
    tunnel: path "C:/Users/anton/Desktop/liquenes/colorlichen2.png" ("File Path") -> [w663]
    tunnel: w68 -> [w666]
    tunnel: w63 -> [w665]
    shift-right: [w663] -> _
    shift-left: _ -> [w664]
    stop <- FALSE continue-if-true
    n207 = First Call?() -> (First Call?: T/F=w662:bool)
    n208 = Not Equal?(x=w664, y=w663) -> (x != y?=w661:bool)
    n209 = Or(x=w661, y=w662) -> (x .or. y?=w660:bool)
    n210 = case shown="True" w660 {
      tunnel: [w673 w686] -> w671
      tunnel: w670 -> [w673 w678]
      tunnel: [w672 w683] -> w668
      tunnel: w667 -> [w672 w677]
      tunnel: w666 -> [_ w682]
      tunnel: w665 -> [_ w679]
      tunnel: w663 -> [_ w675]
      frame False {
      }
      frame True {
        n211 = Call Chain() -> (call chain=w681:string[])
        n212 = stacked-sequence {
          tunnel: w678 -> [w691]
          tunnel: w677 -> [w690]
          tunnel: [w690] -> w676
          tunnel: [w689] -> _
          frame #0 {
            n213 = call "IMAQ Dispose"("Image"=w691) -> ("error out"=w689:errorcluster)  [unwired: 2 in, 3 out]
          }
        }
        n214 = Index Array(array=w681) -> (element=w680:string)  [unwired: 1 in]
        n215 = Format Into String(format string="CL Template %s %s" ("Image Name"), w680, w679) -> (resulting string=w688:string)  [unwired: 2 in, 1 out]
        n216 = call "IMAQ Create"("Image Name"=w688, "Image Type"=w682, "error in (no error)"=w676) -> ("New Image"=w685:T3, "error out"=w684:errorcluster)  [unwired: 1 in, 1 out]
        n217 = call <vilib>:"IVA Get Alternate Path.vi"("Path In"=w675) -> ("Path Out"=w674:path)  [unwired: 10 out]
        n218 = call "IMAQ Read Image And Vision Info"("File Path"=w674, "error in (no error)"=w684, "Image"=w685) -> ("error out"=w683:errorcluster, "Image Out"=w686:T3)  [unwired: 1 in, 6 out]
      }
    }
  }
  n219 = Unbundle By Name("ROI Descriptor (Lichen 2 Cell 6)") -> ("Global Rectangle"=w60:i32[])
  n220 = call "IMAQ Setup Match Color Pattern"("Match Feature Mode"=w72, "error in (no error)"=w58, "Color Sensitivity"=w71, "Search Strategy"=w70) -> ("Match Color Pattern Setup Data"=w62:string, "error out"=w61:errorcluster)  [unwired: 5 in, 5 out]
  n221 = call "IMAQ Match Color Pattern"("Minimum Match Score"=sgl 600.0, "Number of Matches Requested"=1, "Optional Rectangle"=w60, "error in (no error)"=w61, "Match Color Pattern Setup Data"=w62, "Template Image"=w59, "Image"=w65) -> ("error out"=w66:errorcluster, "Number of Matches"=→"Number of Matches (Lichen 2 Cell 6)":i32, "Matches"=w64:T5)  [unwired: 2 out]
  n222 = call <vilib>:"IVA Store Color Location Results.vi"("error in (no error)"=w66, "Matches"=w64, "Step Name"=w63, "Image in"=w65) -> ("error out"=w57:errorcluster, "Image dup"=w50:T3)  [unwired: 6 out]
  n223 = call <vilib>:"IVA Clear Coordsys Errors.vi"("error in (no error)"=w57) -> ("error out"=w56:errorcluster)  [unwired: 10 in]
  n224 = call "IMAQ ColorThreshold"("Blue or Luma or Val or Inten Range"=cluster{"Lower value":i32, "Upper value":i32} {"Lower value"=0, "Upper value"=99}, "Replace Value"=1, "Green or Sat Range"=cluster{"Lower value":i32, "Upper value":i32} {"Lower value"=102, "Upper value"=255}, "Color Mode"=w54, "error in (no error)"=w56, "Red or Hue Range"=cluster{"Lower value":i32, "Upper value":i32} {"Lower value"=0, "Upper value"=239}, "Image Src"=w50) -> ("error out"=w49:errorcluster, "Image Dst Out"=w47:T3)  [unwired: 1 in, 2 out]
  n225 = call "IMAQ FillHole"("error in (no error)"=w49, "Image Src"=w47, "Connectivity 4/8 (8)"=FALSE) -> ("error out"=w46:errorcluster, "Image Dst Out"=w41:T3)  [unwired: 1 in, 2 out]
  n226 = call "IMAQ RemoveParticle"("Connectivity 4/8 (8)"=FALSE, "Low Pass/High Pass (Low)"=FALSE, "Square/Hexa (Square)"=TRUE, "error in (no error)"=w46, "Number of Erosion"=1, "Image Src"=w41) -> ("error out"=w40:errorcluster, "Image Dst Out"=w39:T3)  [unwired: 1 in, 3 out]
  n227 = call <vilib>:"IVA Histogram.vi"("Color Mode"=w37, "error in (no error)"=w40, "ROI Descriptor"=w35, "Image In"=w39) -> ("error out"=w38:errorcluster, "Histograms"=→"Histogram Graph" →"Histogram (Histogram 2)":u32[][], "Image Out"=w34:T3)  [unwired: 5 out]
  n228 = disable-structure "Conditional Disable Structure" shown="TARGET_TYPE==Windows" {
    disable-tunnel: w38 -> [w695 w696]
    disable-tunnel: [w694 w696] -> w32
    disable-tunnel: w34 -> [w693 w697]
    disable-tunnel: [w693 w697] -> w25
    disable-tunnel: u8 0 ("Y Scale.Mapping Mode") -> [w692 _]
    frame condition #0 (active) {
      n229 = property on="Histogram Graph" class="WFGraph (strict)"(error in=w695, "Y Scale.Mapping Mode"=w692) -> (error out=w694:errorcluster)  [unwired: 1 in, 1 out]
    }
    frame condition #1 {
    }
  }
  n230 = call <vilib>:"IVA Clear Coordsys Errors.vi"("error in (no error)"=w32) -> ("error out"=w31:errorcluster)  [unwired: 10 in]
  n231 = call "IMAQ GetFileInfo"("error in (no error)"=w31, "File Path"=w23) -> ("error out"=w21:errorcluster, "Image Type"=w29:T4)  [unwired: 8 out]
  n232 = call "IMAQ ReadFile 2"("Use File Path Image Type"=TRUE, "File Path"=w23, "error in (no error)"=w21, "Image"=w25) -> ("error out"=w22:errorcluster, "Image Out"=w24:T3)  [unwired: 3 in, 3 out]
  n233 = case shown="1, 7" w29 {
    tunnel: w24 -> [w699 w708]
    tunnel: w22 -> [w698 w707]
    tunnel: w28 -> [_ w701]
    tunnel: w27 -> [_ w711]
    tunnel: [w699 w710] -> w14
    tunnel: [w698 w709] -> w26
    frame 0, Default {
    }
    frame 1, 7 {
      n234 = call "IMAQ Image Bit Depth"("Image"=w708, "error in (no error)"=w707, "Get/Set Bit Depth? (Set)"=FALSE) -> ("Image Out"=w705:T3, "Bit Depth"=w704:u32, "error out"=w703:errorcluster)  [unwired: 10 in]
      n235 = Equal To 0?(x=w704) -> (x = 0?=w702:bool)
      n236 = And(x=w702, y=w701) -> (x .and. y?=w700:bool)
      n237 = case shown="True" w700 {
        tunnel: w705 -> [w713 w719]
        tunnel: w703 -> [w712 w718]
        tunnel: w711 -> [_ w717]
        tunnel: [w713 w716] -> w710
        tunnel: [w712 w715] -> w709
        frame False {
        }
        frame True {
          n238 = call "IMAQ Image Bit Depth"("Image"=w719, "Bit Depth (0)"=w717, "error in (no error)"=w718, "Get/Set Bit Depth? (Set)"=TRUE) -> ("Image Out"=w716:T3, "error out"=w715:errorcluster)  [unwired: 9 in, 1 out]
        }
      }
    }
  }
  n239 = call "IMAQ ColorThreshold"("Blue or Luma or Val or Inten Range"=cluster{"Lower value":i32, "Upper value":i32} {"Lower value"=103, "Upper value"=179}, "Replace Value"=1, "Green or Sat Range"=cluster{"Lower value":i32, "Upper value":i32} {"Lower value"=0, "Upper value"=36}, "Color Mode"=w18, "error in (no error)"=w26, "Red or Hue Range"=cluster{"Lower value":i32, "Upper value":i32} {"Lower value"=69, "Upper value"=154}, "Image Src"=w14) -> ("error out"=w13:errorcluster, "Image Dst Out"=w12:T3)  [unwired: 1 in, 2 out]
  n240 = call <vilib>:"IVA Histogram.vi"("Color Mode"=w10, "error in (no error)"=w13, "ROI Descriptor"=w8, "Image In"=w12) -> ("error out"=w11:errorcluster, "Histograms"=→"Histogram Graph 2":u32[][], "Image Out"=w7:T3)  [unwired: 5 out]
  n241 = disable-structure "Conditional Disable Structure" shown="TARGET_TYPE==Windows" {
    disable-tunnel: w11 -> [w723 w724]
    disable-tunnel: [w722 w724] -> w5
    disable-tunnel: w7 -> [w721 w725]
    disable-tunnel: [w721 w725] -> w2
    disable-tunnel: u8 1 ("Y Scale.Mapping Mode") -> [w720 _]
    frame condition #0 (active) {
      n242 = property on="Histogram Graph 2" class="WFGraph (strict)"(error in=w723, "Y Scale.Mapping Mode"=w720) -> (error out=w722:errorcluster)  [unwired: 1 in, 1 out]
    }
    frame condition #1 {
    }
  }
  "Image Out" <- w2
  n243 = call <vilib>:"IVA Clear Coordsys Errors.vi"("error in (no error)"=w5) -> ("error out"=w4:errorcluster)  [unwired: 10 in]
  n244 = property on="Image Out" class="ImageControl"(error in=w4, "Palette:Palette Type"=w1) -> (error out=→"error out":errorcluster)  [unwired: 1 in, 1 out]
